vi "TestStand.GetExecutingStepsAndThreads.vi"(8 "error in (no error)":errorcluster, 11 "Application Manager":refnum<k7>) -> (0 "error out":errorcluster, 1 "Steps":string[][](table), 2 "Threads":string[](array[string]))   [LabVIEW 2019, in "Tools.lvlib"]
uses:
  Tools.lvlib
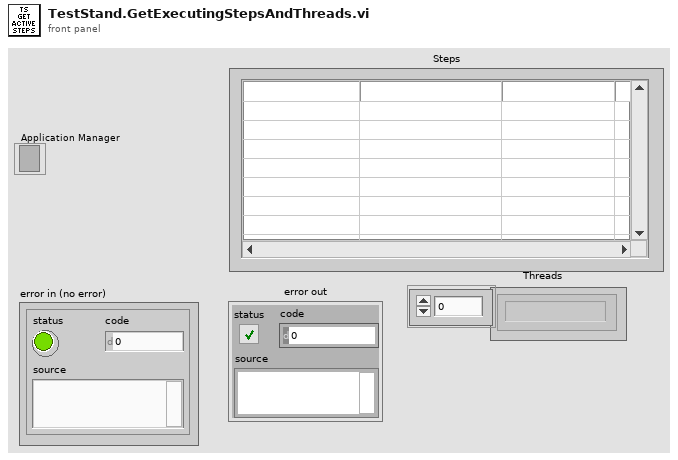
[diagram p1: front panel]
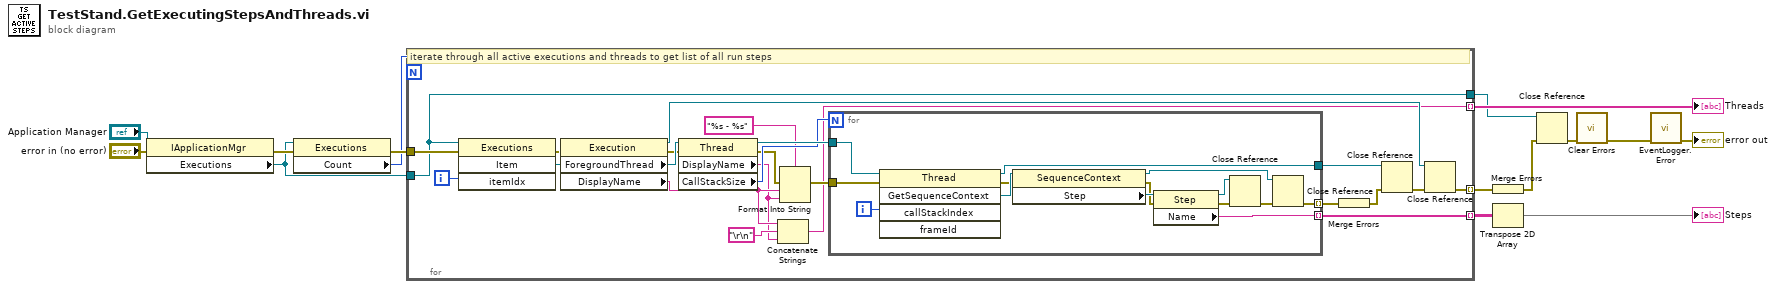
[diagram p0: block diagram]
diagram:
  n1 = property class="IApplicationMgr"(reference="Application Manager", error in="error in (no error)") -> (error out=w10:errorcluster, "Executions"=w8:refnum<k7>)  [unwired: 1 out]
  n2 = property class="Executions"(reference=w8, error in=w10) -> (error out=w11:errorcluster, "Count"=w9:i32)  [unwired: 1 out]
  n3 = for {
    N: w9 -> [_]
    tunnel: w8 -> [w16]
    tunnel: w11 -> [w33]
    tunnel: [w21] -> w12 mode=indexing
    tunnel: [w17] -> w6 mode=indexing
    tunnel: [w28] -> w13 mode=indexing
    tunnel: [w16] -> w2
    i -> [w35]
    # "iterate through all active executions and threads to get list of all run steps"
    n4 = invoke class="Executions" method="Item"(reference=w16, error in=w33, "itemIdx"=w35) -> (error out=w32:errorcluster, "Item"=w34:refnum<k7>)  [unwired: 1 in, 2 out]
    n5 = property class="Execution"(reference=w34, error in=w32) -> (reference out=w22:refnum<k7>, error out=w31:errorcluster, "ForegroundThread"=w37:refnum<k7>, "DisplayName"=w20:string)
    n6 = property class="Thread"(reference=w37, error in=w31) -> (reference out=w38:refnum<k7>, error out=w27:errorcluster, "DisplayName"=w18:string, "CallStackSize"=w36:i32)
    n7 = Concatenate Strings(w20, "\r\n", w18) -> (w17:string)
    n8 = Format Into String(format string="%s - %s", error in=w27, w20, w18) -> (error out=w26:errorcluster)  [unwired: 1 in, 1 out]
    n9 = for {
      N: w36 -> [_]
      tunnel: w38 -> [w52]
      tunnel: [w49] -> w28 mode=indexing
      tunnel: [w47] -> w25
      tunnel: w26 -> [w46]
      tunnel: [w39] -> w30 mode=indexing
      i -> [w48]
      n10 = invoke class="Thread" method="GetSequenceContext"(reference=w52, error in=w46, "callStackIndex"=w48) -> (reference out=w47:refnum<k7>, error out=w45:errorcluster, "GetSequenceContext"=w51:refnum<k7>)  [unwired: 2 in, 2 out]
      n11 = property class="SequenceContext"(reference=w51, error in=w45) -> (reference out=w41:refnum<k7>, error out=w44:errorcluster, "Step"=w50:refnum<k7>)
      n12 = property class="Step"(reference=w50, error in=w44) -> (reference out=w43:refnum<k7>, error out=w42:errorcluster, "Name"=w49:string)
      n13 = Close Reference(reference=w43, error in (no error)=w42) -> (error out=w40:errorcluster)
      n14 = Close Reference(reference=w41, error in (no error)=w40) -> (error out=w39:errorcluster)
    }
    n15 = Merge Errors(w30) -> (w24:errorcluster)
    n16 = Close Reference(reference=w25, error in (no error)=w24) -> (error out=w23:errorcluster)
    n17 = Close Reference(reference=w22, error in (no error)=w23) -> (error out=w21:errorcluster)
  }
  "Threads" <- w6
  n18 = Merge Errors(w12) -> (w5:errorcluster)
  n19 = Transpose 2D Array(2D array=w13) -> (transposed array=→"Steps":string[][])
  n20 = Close Reference(reference=w2, error in (no error)=w5) -> (error out=w4:errorcluster)
  n21 = call <vilib>:"Clear Errors.vi"("error in (no error)"=w4) -> ("error out"=w1:errorcluster)  [unwired: 5 in, 1 out]
  n22 = call "EventLogger.Error.vi"("error in"=w1) -> ("error out"=→"error out":errorcluster)  [unwired: 10 in]
